vi "GUI Controller_Create.vi"(0 "reference in":refnum<class "GUI Controller.lvclass">, 5 "error in (no error)":errorcluster) -> (14 "reference out":refnum<class "GUI Controller.lvclass">, 19 "error out":errorcluster)   [LabVIEW 2015, in "GUI Controller.lvclass"]
doc: "Constructor."
uses:
  GUI Controller.lvclass
  <vilib>/addons/_AddQ/G#Object/G#Object.lvclass
  Project Panels_class/Project Panels.lvclass
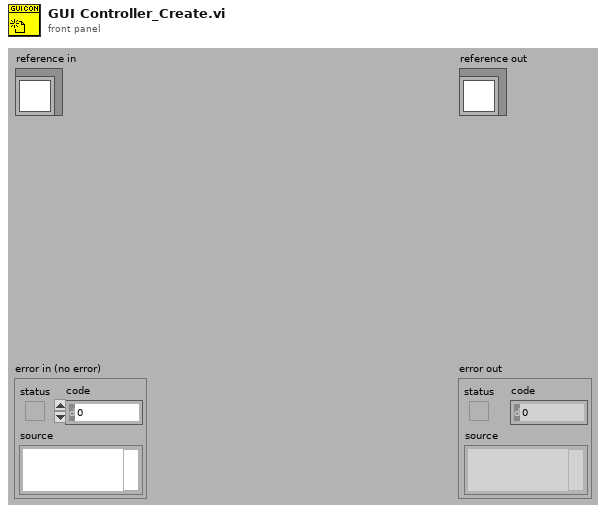
[diagram p1: front panel]
types:
  T1 = typedef "GUI Controller.lvclass/ObjectAttributesRef.ctl" = refnum<data-value>
  T2 = typedef "GUI Controller.lvclass/ObjectAttributes.ctl" = cluster{"MyAttribute":dbl, "state":T3, "project_panels_ref":refnum<class "Project Panels.lvclass">, "items_controller_ref":refnum<class "Items Controller.lvclass">, "notification_controller_ref":refnum<class "Notification Controller.lvclass">, "partstracking_controller_ref":refnum<class "PartsTracking Controller.lvclass">, "file_controller_ref":refnum<class "File Controller.lvclass">, "low_resolution?":bool}
  T3 = typedef "GUI Controller.lvclass/state.ctl" = enum16{"initiate", "checkNotificationItems", "checkNotificationTracking", "operate", "updateFromFile", "stop"}
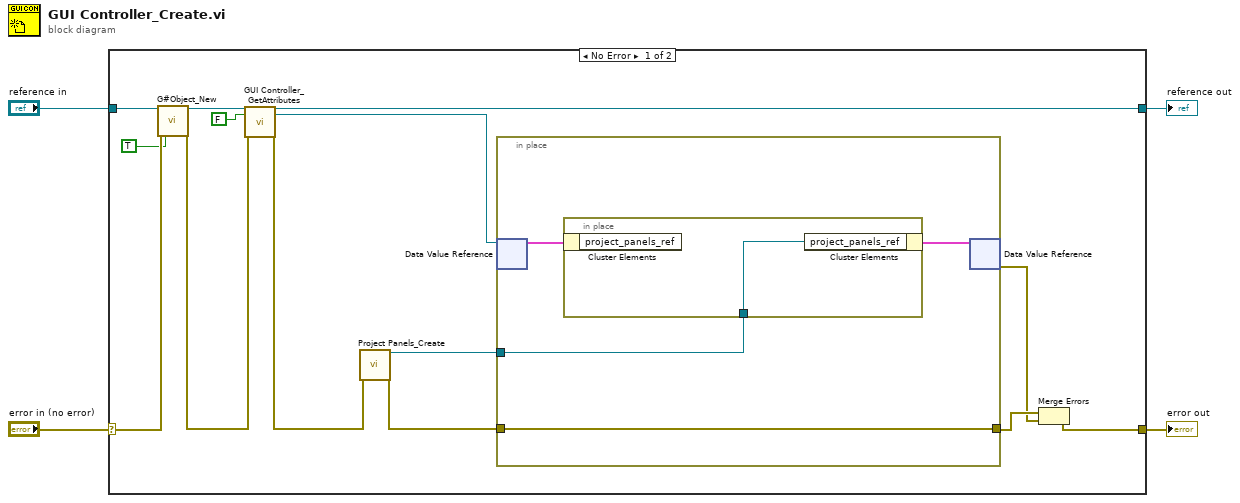
[diagram p0: block diagram]
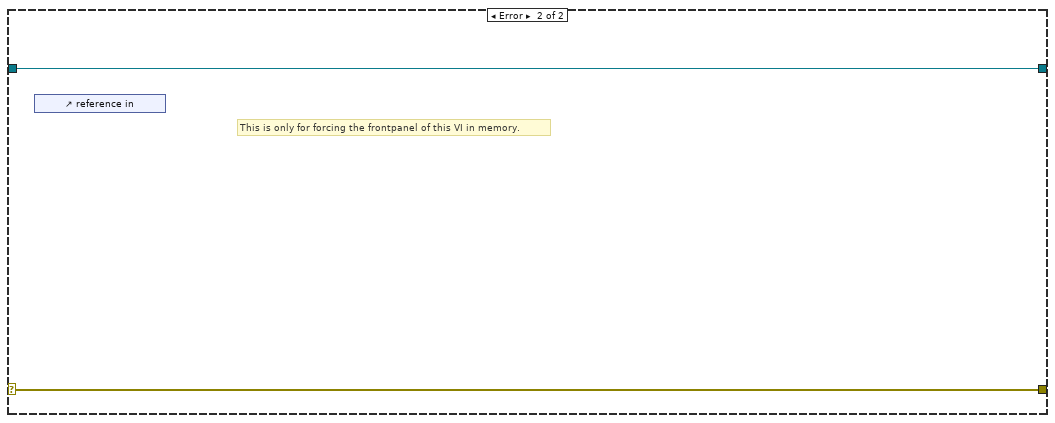
[diagram p2: hidden frame]
diagram:
  n1 = case shown="No Error" "error in (no error)" {
    selector: "error in (no error)" -> [w17 w25]
    tunnel: [w16 w25] -> w3
    tunnel: [w11 w24] -> w1
    tunnel: "reference in" -> [w18 w24]
    frame No Error {
      n2 = call <vilib>:"G#Object_New.vi"("reference in"=w18, "error in (no error)"=w17, "user counter (T)?"=TRUE ("User Counter")) -> ("reference out"=w12:refnum<class "GUI Controller.lvclass">, "error out"=w10:errorcluster)  [unwired: 14 in, 1 out]
      n3 = call "GUI Controller_GetAttributes.vi"("reference in"=w12, "return data? (T)"=FALSE ("return data"), "error in (no error)"=w10) -> ("reference out"=w11:refnum<class "GUI Controller.lvclass">, "attributes ref"=w9:T1, "error out"=w7:errorcluster)  [unwired: 13 in, 1 out]
      n4 = call "Project Panels_Create.vi"("error in (no error)"=w7) -> ("reference out"=w5:refnum<class "Project Panels.lvclass">, "error out"=w6:errorcluster)  [unwired: 17 in]
      n5 = in-place {
        in-place-border: w6 -> [w20]
        in-place-border: [w20] -> w14
        in-place-border: w5 -> [w19]
        n6 = in-place-dvr #1(w9) -> (w21:T2)  [unwired: 1 out]
        n7 = in-place {
          in-place-border: w19 -> [w23]
          n8 = in-place-cluster #2(w21) -> ()  [unwired: 1 out]
          n9 = in-place-cluster #2("project_panels_ref"=w23) -> (w22:T2)
        }
        n10 = in-place-dvr #1(w22) -> (w13:errorcluster)  [unwired: 1 out]
      }
      n11 = Merge Errors(w14, w13) -> (w16:errorcluster)
    }
    frame Error {
      # "This is only for forcing the frontpanel of this VI in memory."
      n12 = control-ref of="reference in"() -> ()  [unwired: 1 out]
    }
  }
  "error out" <- w3
  "reference out" <- w1
